vi "Final Project GUI.vi"() -> ()   [LabVIEW 2021]
uses:
  Serial - XON-XOFF Characters.ctl
  Serial - ASCII Characters-1.ctl
  Serial - Settings.ctl
  Lab4/ESP32-PSOC-State Machine.ctl
  <vilib>/Instr/_visa.llb/VISA Flush IO Buffer Mask.ctl
  <vilib>/numeric/Random Number (Range) DBL.vi
  <vilib>/addons/control/pid/pid.llb/PID (DBL).vi
  <vilib>/Instr/_visa.llb/VISA Configure Serial Port (Instr).vi
  <vilib>/picture/picture.llb/Draw True-Color Pixmap.vi
  <vilib>/addons/control/pid/NI_PID_pid.lvlib
  <vilib>/Analysis/NI_AALBase.lvlib
panel:
  out "Actuator Test Chart 4":dbl(graph)
  out "Actuator Test Chart 3":dbl(graph)
  out "Actuator Test Chart 2":dbl(graph)
  in  "Stop 7":bool
  in  "Stop 6":bool
  in  "Stop 5":bool
  out "Actuator Length (inches) 4":string
  out "Actuator Length (inches) 3":string
  out "Actuator Length (inches) 2":string
  out "Actuator Length (inches)":string
  out "Actuator Test Chart":dbl(graph)
  in  "Stop 4":bool
  in  "Termination Character 2":u8=13 format="%.0x"
  in  "End Write on Termination Character? 2":bool=TRUE
  in  "VISA resource name 2":refnum<visa-resource-name>="COM7"
  in  "XON/XOFF Characters 2":T1={"XON"=enum."DC1", "XOFF"=enum."DC3"}
  in  "Serial Settings 2":T3={"baud rate"=115200, "data bits"=8, "parity"=enum."None", "stop bits"=10, "flow control"=0} {"flow control" items=["None"=0, "XON/XOFF"=1, "RTS/CTS"=2, "DTR/DSR"=4]; "stop bits" items=["1.0"=10, "1.5"=15, "2.0"=20]; "data bits" min=5 max=8 step=1; "baud rate" items=["75"=75, "110"=110, "134"=134, "150"=150, "300"=300, "600"=600, "1200"=1200, "1800"=1800, "2400"=2400, "4800"=4800, "7200"=7200, "9600"=9600, "14400"=14400, "19200"=19200, "28800"=28800, "38400"=38400, "56000"=56000, "57600"=57600, "115200"=115200, "128000"=128000, "230400"=230400]}
  in  "End Read on Termination Character? 2":bool=TRUE
  out "Response 3":string
  out "Temperature (deg C)":dbl(graph)
  out "Temperature Histogram":T4(graph)
  in  "Command":string="\n\n"
  in  "Stop 3":bool
  in  "Write":bool
  out "String":string
  out "Response 2":string
  in  "Toggle LED":bool
  in  "Command A":bool
  in  "Command B":bool
  in  "Enum":T5
  out "Connected":bool
  out "error":bool
  out "Read Count":u32=1000
  out "Response":string
  out "Serial Settings:Number of Bytes at Serial Port":u32
  in  "End Read on Termination Character?":bool=TRUE
  in  "Serial Settings":T3={"baud rate"=115200, "data bits"=8, "parity"=enum."None", "stop bits"=10, "flow control"=0} {"flow control" items=["None"=0, "XON/XOFF"=1, "RTS/CTS"=2, "DTR/DSR"=4]; "stop bits" items=["1.0"=10, "1.5"=15, "2.0"=20]; "data bits" min=5 max=8 step=1; "baud rate" items=["75"=75, "110"=110, "134"=134, "150"=150, "300"=300, "600"=600, "1200"=1200, "1800"=1800, "2400"=2400, "4800"=4800, "7200"=7200, "9600"=9600, "14400"=14400, "19200"=19200, "28800"=28800, "38400"=38400, "56000"=56000, "57600"=57600, "115200"=115200, "128000"=128000, "230400"=230400]}
  in  "XON/XOFF Characters":T1={"XON"=enum."DC1", "XOFF"=enum."DC3"}
  in  "VISA resource name":refnum<visa-resource-name>="COM7"
  in  "End Write on Termination Character?":bool=TRUE
  in  "Termination Character":u8=10 format="%.0x"
  in  "Stop 2":bool
  out "Waveform Chart 2":dbl(graph)
  out "Waveform Chart":dbl(graph)
  in  "PID gains":T6={"proportional gain (Kc)"=20.0, "integral time (Ti, min)"=0.008, "derivative time (Td, min)"=0.001} {"derivative time (Td, min)" format="%.3f"; "integral time (Ti, min)" format="%.3f"; "proportional gain (Kc)" format="%.3f"}
  out "2D Picture 2":picture
  out "24-bit pixmap":u32[][](array[numeric]) format="%x"
  out "2D Picture":picture
  in  "Stop":bool
  # "Overview: Demonstrates the use of the VISA functions to write commands to and read responses from a serial instrument continuously in a loop.\nRequirements: NI-VISA Driver\nInstructions:\n1. Using Windows Device Manager take note of the COM port given by Windows to your microcontroller connection\n2. Change the VISA resource name to your COM port from step 1\n3. Run the VI.\n4. Press reset on your microcontroller\n5. Wait for the Ready to accept  Commands message\n6. The sample program response to Command :  T, A, B, I\n7. Specify a Command and click the Write button.\n8 The corresponding response should appear in the Response Window\n9. Click Stop to stop the VI."
  # "CAR"
  # "BONUS ADDITIONS (if time allows)"
types:
  T1 = typedef "Serial - XON-XOFF Characters.ctl" = cluster{"XON":T2, "XOFF":T2}
  T2 = typedef "Serial - ASCII Characters-1.ctl" = enum16{"NUL", "SOH", "STX", "ETX", "EOT", "ENQ", "ACK", "BEL", "BS", "HT", "LF", "VT", "FF", "CR", "SO", "SI", "DLE", "DC1", "DC2", "DC3", "DC4", "NAK", "SYN", "ETB", "CAN", "EM", "SUB", "ESC", "FS", "GS", "RS", "US", "SP", "!", "\"", "#", "$", "%", "&", "'", "(", ")", "*", "+", ",", "- (-)", ".", "/", "0", "1", "2", "3", "4", "5", "6", "7", "8", "9", ":", ";", "<", "=", ">", "?", "@", "A", "B", "C", "D", "E", "F", "G", "H", "I", "J", "K", "L", "M", "N", "O", "P", "Q", "R", "S", "T", "U", "V", "W", "X", "Y", "Z", "[", "\\", "]", "^", "_", "`", "a", "b", "c", "d", "e", "f", "g", "h", "i", "j", "k", "l", "m", "n", "o", "p", "q", "r", "s", "t", "u", "v", "w", "x", "y", "z", "{", "|", "}", "~"}
  T3 = typedef "Serial - Settings.ctl" = cluster{"baud rate":u32, "data bits":u16, "parity":enum16{"None", "Odd", "Even", "Mark", "Space"}, "stop bits":u16, "flow control":u16}
  T4 = cluster{"X Values":dbl[], "Histogram: h(x)":i32[]}
  T5 = typedef "ESP32-PSOC-State Machine.ctl" = enum8{"Init", "Connect", "idle", "send", "wait", "receive", "que", "error", "exit"}
  T6 = cluster{"proportional gain (Kc)":dbl, "integral time (Ti, min)":dbl, "derivative time (Td, min)":dbl}
  T7 = typedef "VISA Flush IO Buffer Mask.ctl" = u16
  T8 = typedef "imagedata.ctl" = cluster{"image type":i32, "image depth":i32, "image":u8[], "mask":u8[], "colors":u32[], "Rectangle":cluster{"left":i16, "top":i16, "right":i16, "bottom":i16}}
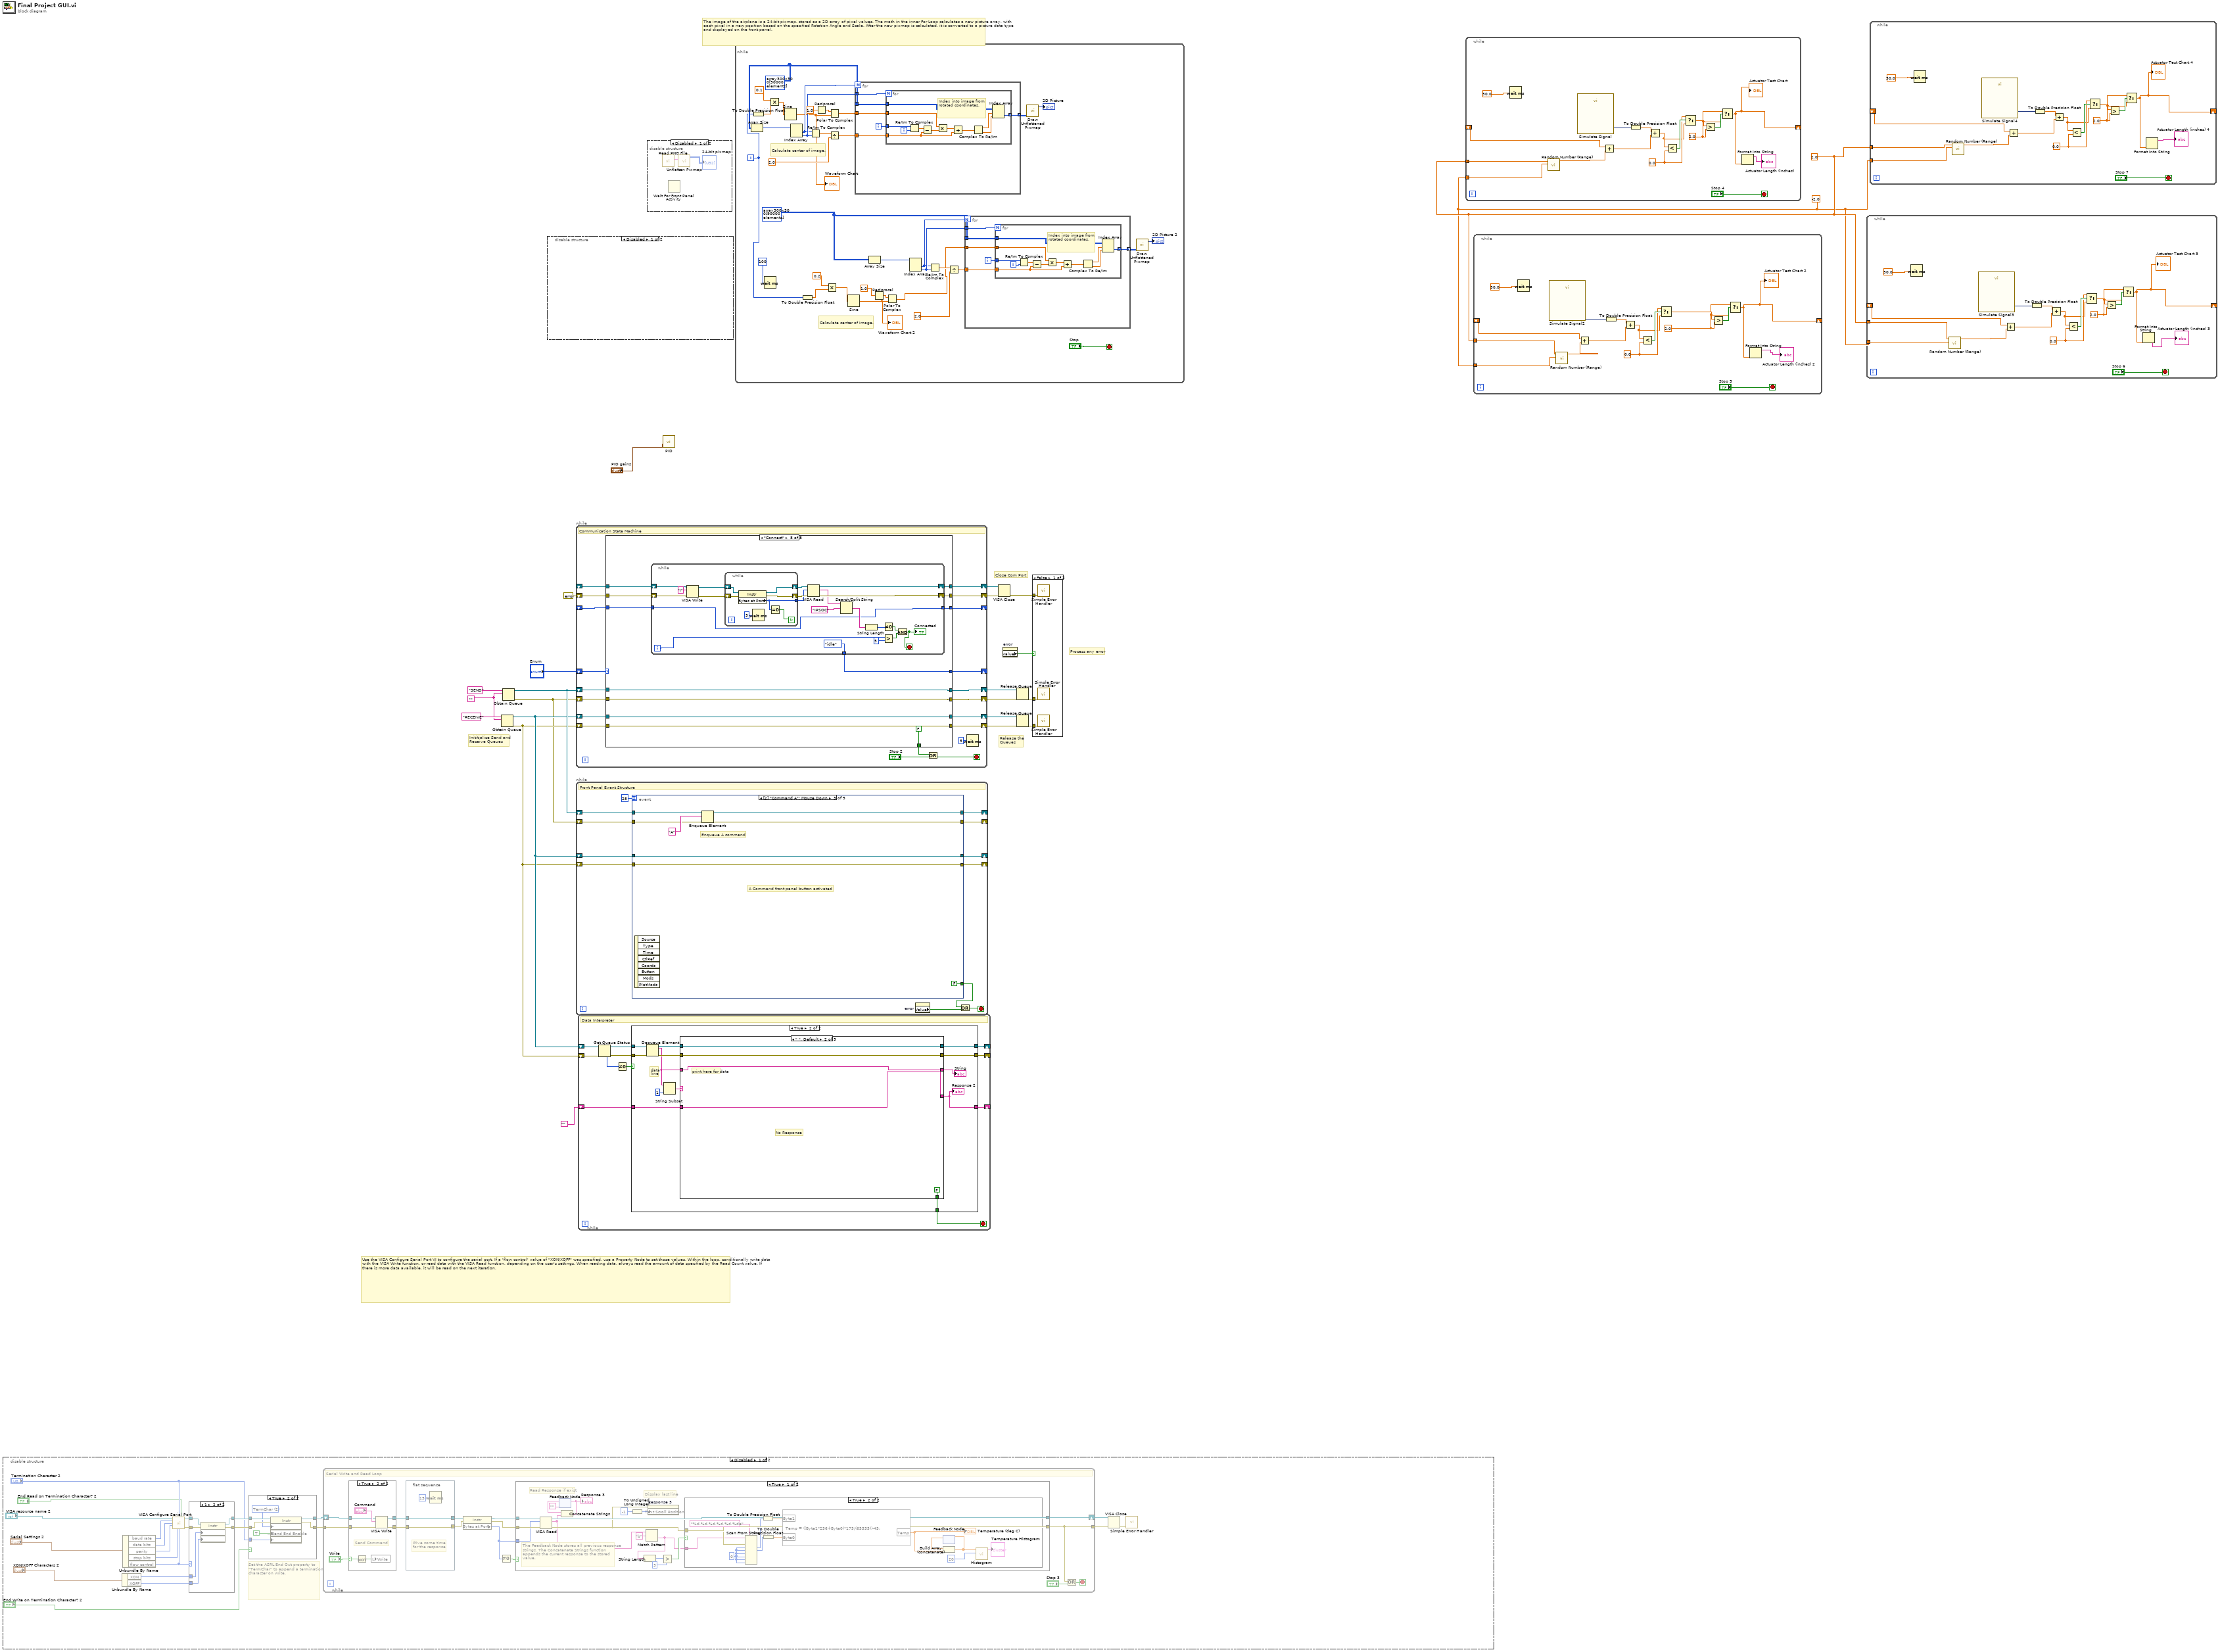
[diagram p0: block diagram]
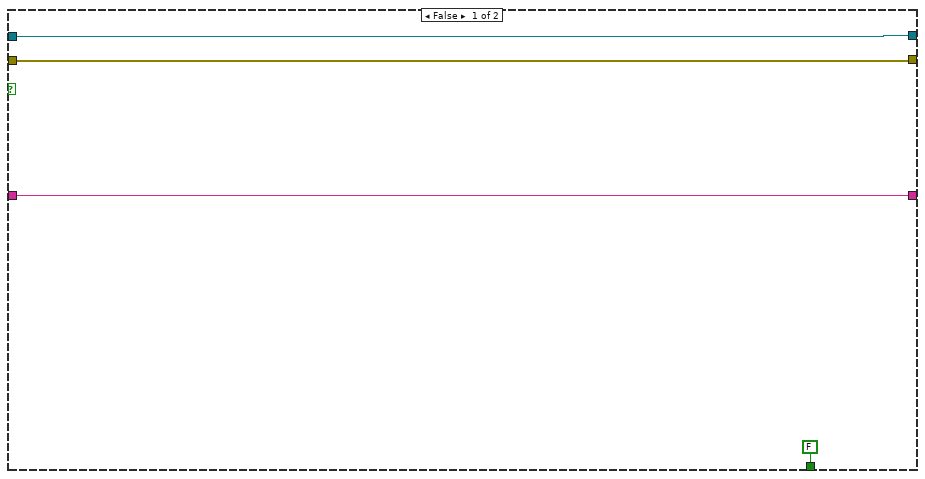
[diagram p9: hidden frame]
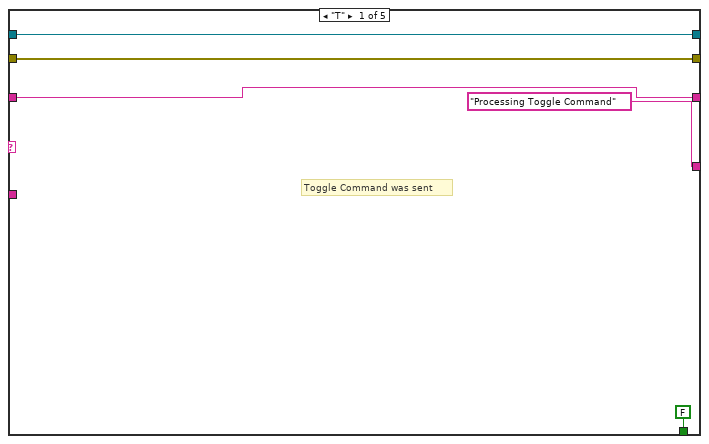
[diagram p10: hidden frame]
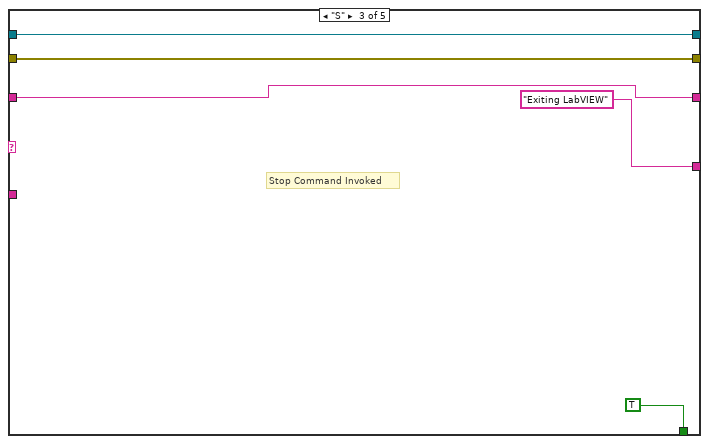
[diagram p11: hidden frame]
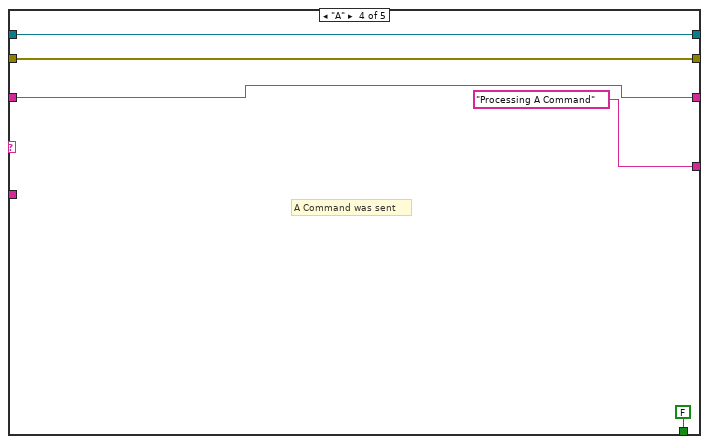
[diagram p12: hidden frame]
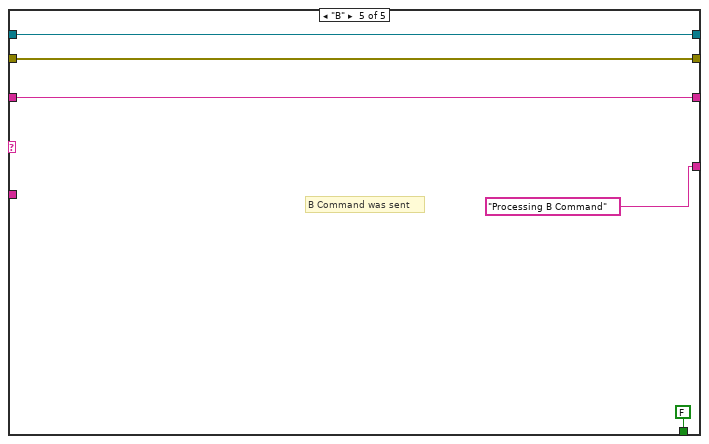
[diagram p13: hidden frame]
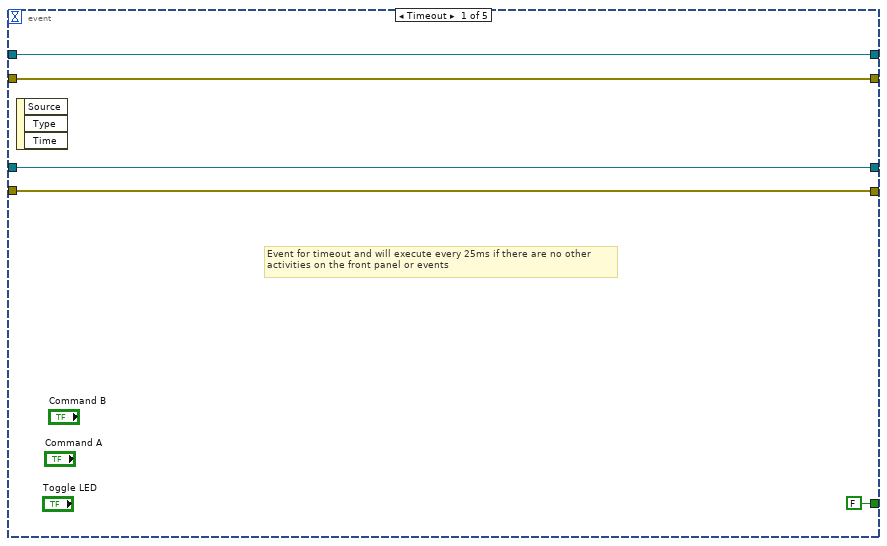
[diagram p14: hidden frame]
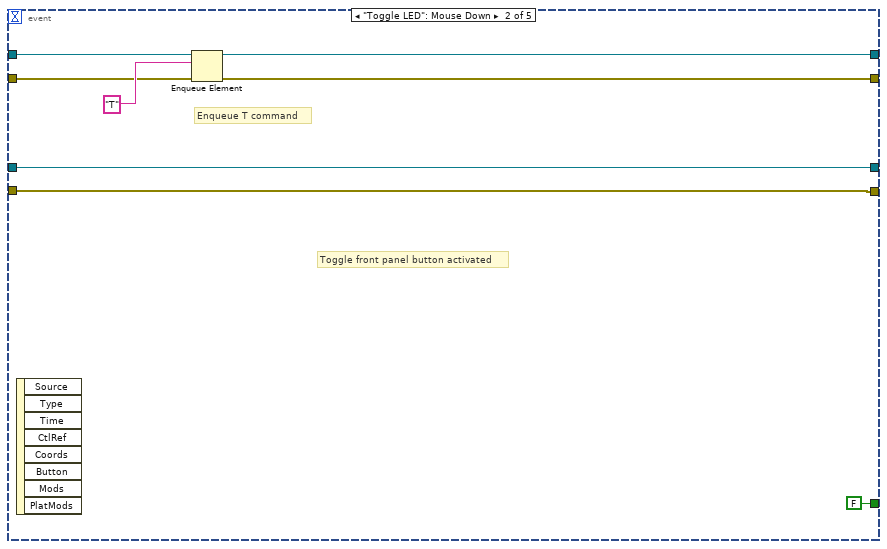
[diagram p15: hidden frame]
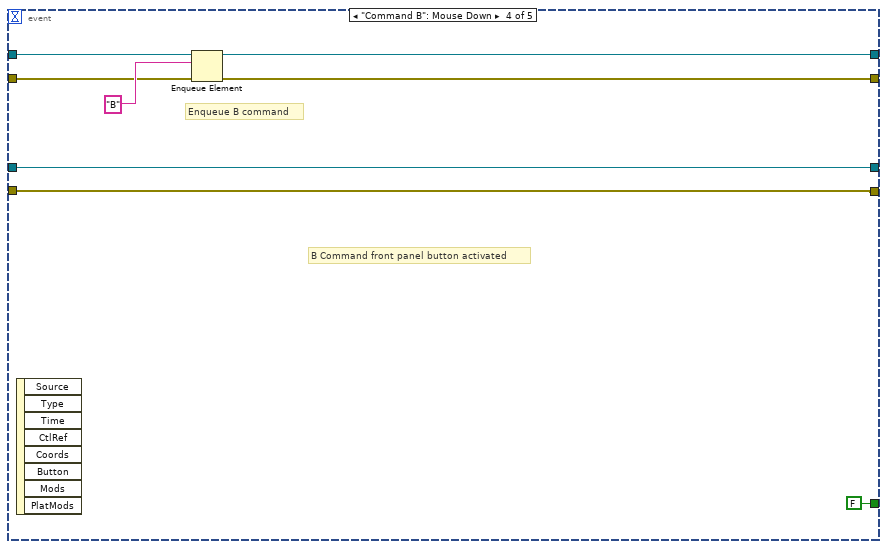
[diagram p16: hidden frame]
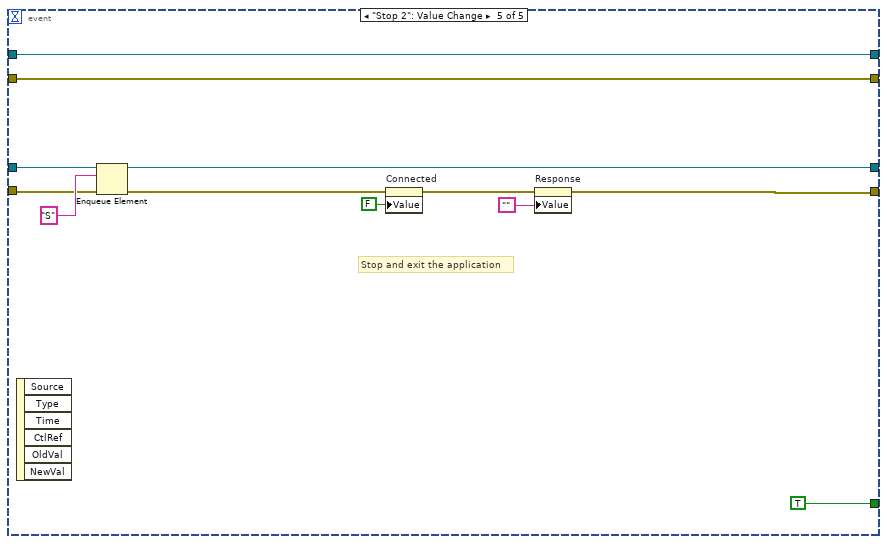
[diagram p17: hidden frame]
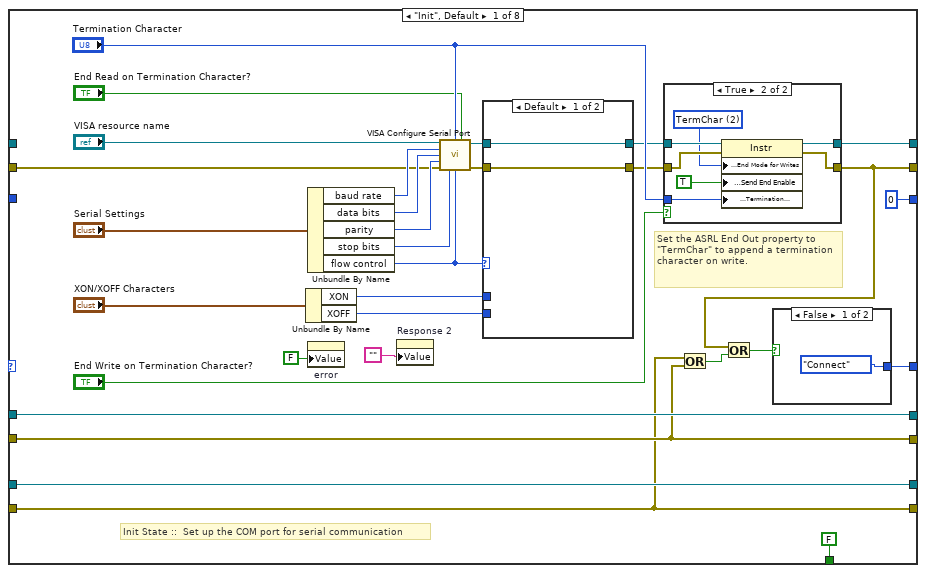
[diagram p18: hidden frame]
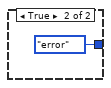
[diagram p19: hidden frame]
diagram:
  w2 = 2.0
  w1 = -2.0
  w12 = ""
  # "Use the VISA Configure Serial Port VI to configure the serial port. If a 'flow control' value of \"XON/XOFF\" was specified, use a Property Node to set those values. Within the loop, conditionally write data with the VISA Write function, or read data with the VISA Read function, depending on the user's settings. When reading data, always read the amount of data specified by the Read Count value. If there is more data available, it will be read on the next iteration."
  # "Process any error"
  # "Release the\nQueues"
  # "Close Com Port"
  # "Inititialize Send and\nReceive Queues"
  # "The image of the airplane is a 24-bit pixmap, stored as a 2D array of pixel values. The math in the inner For Loop calculates a new picture array, with each pixel in a new position based on the specified Rotation Angle and Scale. After the new pixmap is calculated, it is converted to a picture data type and displayed on the front panel."
  n1 = disable-structure shown="Disabled" {
    frame Disabled {
      # "Set the ASRL End Out property to \"TermChar\" to append a termination character on write."
      n2 = Unbundle By Name("XON/XOFF Characters 2") -> ("XON"=w35:T2, "XOFF"=w34:T2)
      n3 = Unbundle By Name("Serial Settings 2") -> ("baud rate"=w40:u32, "data bits"=w41:u16, "parity"=w42:enum16{"None", "Odd", "Even", "Mark", "Space"}, "stop bits"=w43:u16, "flow control"=w36:u16)
      n4 = call-poly "VISA Configure Serial Port"("VISA resource name"="VISA resource name 2", "termination char\n(0xA = '\\n' = LF)"="Termination Character 2", "Enable Termination\nChar (T)"="End Read on Termination Character? 2", "baud rate (9600)"=w40, "data bits (8)"=w41, "parity (0:none)"=w42, "stop bits (10: 1 bit)"=w43, "flow control (0:none)"=w36) -> ("VISA resource name out"=w44:refnum<visa-resource-name>, "error out"=w45:errorcluster)  [unwired: 2 in, 4 out]
      n5 = case shown="1" w36 {
        tunnel: [w55 w62] -> w33
        tunnel: [w56 w61] -> w31
        tunnel: w45 -> [w55 w60]
        tunnel: w44 -> [w56 w59]
        tunnel: w35 -> [_ w58]
        tunnel: w34 -> [_ w57]
        frame Default {
        }
        frame 1 {
          n6 = property class="Instr"(reference=w59, error in=w60, "Serial Settings:Flow Control XON Character"=w58, "Serial Settings:Flow Control XOFF Character"=w57) -> (reference out=w61:refnum<visa-resource-name>, error out=w62:errorcluster)
        }
      }
      n7 = case shown="True" "End Write on Termination Character? 2" {
        tunnel: w31 -> [w46 w54]
        tunnel: w33 -> [w47 w53]
        tunnel: [w46 w52] -> w30
        tunnel: [w47 w51] -> w32
        tunnel: "Termination Character 2" -> [_ w49]
        frame False {
        }
        frame True {
          w50 = u16 2 items=["None", "LastBit", "TermChar", "Break"] ("Serial Settings:Serial End Mode for Writes")
          n8 = property class="Instr"(reference=w54, error in=w53, "Serial Settings:End Mode for Writes"=w50, "Message Based Settings:Send End Enable"=TRUE, "Message Based Settings:Termination Character"=w49) -> (reference out=w52:refnum<visa-resource-name>, error out=w51:errorcluster)
        }
      }
      n9 = while {
        shift-right: [w77] -> w37
        shift-left: w30 -> [w76]
        tunnel: w32 -> [w75]
        tunnel: [w73] -> w38
        stop <- w74 stop-if-true
        # "Serial Write and Read Loop"
        n10 = case shown="True" "Write" {
          selector: "Write" -> [_ w84]
          tunnel: w76 -> [w82 w88]
          tunnel: w75 -> [w81 w87]
          tunnel: [w82 w86] -> w66
          tunnel: [w81 w85] -> w64
          frame False {
          }
          frame True {
            # "Send Command"
            n11 = Not(x=w84) -> (.not. x?=w83:bool)
            n12 = local write "Write"(w83) -> ()
            n13 = VISA Write(VISA resource name=w88, write buffer="Command", error in (no error)=w87) -> (VISA resource name out=w86:refnum<visa-resource-name>, error out=w85:errorcluster)  [unwired: 1 out]
          }
        }
        n14 = flat-sequence {
          tunnel: w66 -> [w80]
          tunnel: [w80] -> w65
          tunnel: w64 -> [w79]
          tunnel: [w79] -> w63
          frame #0 {
            # "Give some time\nfor the response"
            n15 = Wait (ms)(milliseconds to wait=u32 15) -> ()  [unwired: 1 out]
          }
        }
        n16 = property class="Instr"(reference=w65, error in=w63) -> (reference out=w69:refnum<visa-resource-name>, error out=w70:errorcluster, "Bytes at Port"=w67:u32)
        n17 = Not Equal To 0?(x=w67) -> (x != 0?=w68:bool)
        n18 = case shown="True" w68 {
          tunnel: [w99 w120] -> w77
          tunnel: w69 -> [w105 w120]
          tunnel: [w96 w119] -> w73
          tunnel: w70 -> [w104 w119]
          tunnel: w67 -> [w100 _]
          frame True {
            # "Read Response if exist"
            # "Display last line"
            # "The Feedback Node stores all previous response strings. The Concatenate Strings function appends the current response to the stored value."
            n19 = VISA Read(VISA resource name=w105, byte count=w100, error in (no error)=w104) -> (VISA resource name out=w99:refnum<visa-resource-name>, read buffer=w91:string, error out=w96:errorcluster)  [unwired: 1 out]
            n20 = feedback #1("") -> (w103:string)
            n21 = Concatenate Strings(w103, w91) -> (w102:string)
            "Response 3" <- w102
            n22 = feedback-in #1(w102) -> ()
            n23 = To Unsigned Long Integer(number=-1 ("Text.Scroll Position")) -> (unsigned 32bit integer=w97:u32)
            n24 = Match Pattern(string=w91, regular expression="b") -> (after substring=w90:string)  [unwired: 1 in, 3 out]
            n25 = String Length(string=w90) -> (length=w95:i32)
            n26 = property on="Response 3" class="Str"(error in=w96, "Text.Scroll Position"=w97) -> ()  [unwired: 1 in, 2 out]
            n27 = Greater?(x=w95, y=3) -> (0:w93:bool)
            n28 = case shown="True" w93 {
              tunnel: w96 -> [_ w117]
              tunnel: w90 -> [_ w115]
              frame False {
              }
              frame True {
                w118 = u8 0
                n29 = Scan From String(format string="%d,%d,%d,%d,%d,%de", input string=w115, error in=w117, default 1=w118, default 2=w118, default 3=w118, default 4=w118, default 5=w118, default 6=w118) -> (output 1=w114:u8, output 2=w113:u8)  [unwired: 5 in, 3 out]
                n30 = To Double Precision Float(number=w114) -> (double precision float=w112:dbl)
                n31 = To Double Precision Float(number=w113) -> (double precision float=w111:dbl)
                n32 = formula code="Temp = ((Byte1*256+Byte0)*175/(65535))-45;"("Byte1"=w112, "Byte0"=w111) -> ("Temp"=w110:dbl)
                "Temperature (deg C)" <- w110
                n33 = feedback #2() -> (w108:dbl[])  [unwired: 1 in]
                n34 = Build Array (concatenate)(w108, w110) -> (w109:dbl[])
                n35 = feedback-in #2(w109) -> ()
                n36 = call <vilib>:"Histogram.vi"("intervals"=20, "X"=w109) -> ("Histogram Graph"=→"Temperature Histogram":T4)  [unwired: 6 in, 3 out]
              }
            }
          }
          frame False {
          }
        }
        n37 = Or(x=w73, y="Stop 3") -> (x .or. y?=w74:bool)
      }
      n38 = VISA Close(VISA resource name=w37, error in (no error)=w38) -> (error out=w39:errorcluster)
      n39 = call <vilib>:"Simple Error Handler.vi"("error in (no error)"=w39) -> ()  [unwired: 1 in, 8 out]
    }
    frame Enabled {
    }
  }
  n40 = Obtain Queue(name (unnamed)="RECEIVE", element data type=w12) -> (queue out=w11:refnum<queue>, error out=w10:errorcluster)  [unwired: 3 in, 1 out]
  n41 = Obtain Queue(name (unnamed)="SEND", element data type=w12) -> (queue out=w14:refnum<queue>, error out=w4:errorcluster)  [unwired: 3 in, 1 out]
  n42 = disable-structure shown="Disabled" {
    frame Disabled {
    }
    frame Enabled {
    }
  }
  n43 = while {
    shift-right: [w132] -> w22
    shift-left: w14 -> [w140]
    shift-right: [w131] -> w20
    shift-left: w4 -> [w139]
    shift-right: [w130] -> w21
    shift-left: w11 -> [w138]
    shift-right: [w129] -> w17
    shift-left: w10 -> [w137]
    shift-right: [w124] -> _
    shift-left: "Enum" -> [w123]
    shift-right: [w136] -> w16
    shift-left: _ -> [w133]
    shift-right: [w135] -> w15
    shift-left: errorcluster {"status"=FALSE, "code"=0, "source"=""} ("error out") -> [w134]
    shift-right: [w128] -> _
    shift-left: _ -> [w127]
    stop <- w122 stop-if-true
    # "Communication State Machine"
    n44 = case shown="\"Connect\"" w123 {
      selector: w123 -> [_ _ _ _ _ _ w324 _]
      tunnel: [w170 w206 w237 w250 w283 w308 w323 w333] -> w132
      tunnel: [w144 w196 w225 w244 w263 w305 w322 w332] -> w131
      tunnel: [w150 w204 w227 w254 w284 ESP32-PSOC-State_Machine."exit" ("Enum") w324 w329] -> w124
      tunnel: w140 -> [w170 w208 w239 w250 w283 w308 w323 w333]
      tunnel: w139 -> [w144 w207 w238 w244 w263 w305 w322 w332]
      tunnel: w138 -> [w171 w202 w234 w247 w278 w307 w321 w331]
      tunnel: w137 -> [w143 w195 w224 w243 w262 w304 w312 w330]
      tunnel: [w152 w199 w235 w252 w273 w310 w327 w336] -> w136
      tunnel: [w146 w197 w226 w245 w264 w306 w326 w337] -> w135
      tunnel: w134 -> [w148 w198 w230 w251 w266 w306 w326 w338]
      tunnel: w133 -> [_ w200 w232 w253 w281 w310 w327 w339]
      tunnel: [w171 w202 w234 w247 w276 w307 w319 w331] -> w130
      tunnel: [w143 w195 w224 w243 w277 w304 w315 w330] -> w129
      tunnel: [u32 0 ("Bytes at Port") w201 w233 w249 w279 w309 w325 w334] -> w128
      tunnel: w127 -> [_ w201 w233 _ w275 w309 w325 w335]
      tunnel: [FALSE FALSE FALSE FALSE FALSE FALSE TRUE FALSE] -> w121
      frame "Init", Default {
        # "Init State ::  Set up the COM port for serial communication"
        # "Set the ASRL End Out property to \"TermChar\" to append a termination character on write."
        n45 = Unbundle By Name("XON/XOFF Characters") -> ("XON"=w164:T2, "XOFF"=w165:T2)
        n46 = Unbundle By Name("Serial Settings") -> ("baud rate"=w160:u32, "data bits"=w159:u16, "parity"=w158:enum16{"None", "Odd", "Even", "Mark", "Space"}, "stop bits"=w157:u16, "flow control"=w163:u16)
        n47 = property on="error" class="Bool (strict)"("Value"=FALSE ("error")) -> ()  [unwired: 2 in, 2 out]
        n48 = property on="Response 2" class="Str"("Value"="") -> ()  [unwired: 2 in, 2 out]
        n49 = call-poly "VISA Configure Serial Port"("VISA resource name"="VISA resource name", "termination char\n(0xA = '\\n' = LF)"="Termination Character", "Enable Termination\nChar (T)"="End Read on Termination Character?", "baud rate (9600)"=w160, "data bits (8)"=w159, "parity (0:none)"=w158, "error in (no error)"=w148, "stop bits (10: 1 bit)"=w157, "flow control (0:none)"=w163) -> ("VISA resource name out"=w156:refnum<visa-resource-name>, "error out"=w155:errorcluster)  [unwired: 1 in, 4 out]
        n50 = case shown="Default" w163 {
          tunnel: [w183 w192] -> w166
          tunnel: [w184 w191] -> w167
          tunnel: w155 -> [w183 w190]
          tunnel: w156 -> [w184 w189]
          tunnel: w164 -> [_ w188]
          tunnel: w165 -> [_ w187]
          frame Default {
          }
          frame 1 {
            n51 = To Unsigned Byte Integer(number=w187) -> (unsigned 8bit integer=w186:u8)
            n52 = To Unsigned Byte Integer(number=w188) -> (unsigned 8bit integer=w185:u8)
            n53 = property class="Instr"(reference=w189, error in=w190, "Serial Settings:Flow Control XON Character"=w185, "Serial Settings:Flow Control XOFF Character"=w186) -> (reference out=w191:refnum<visa-resource-name>, error out=w192:errorcluster)
          }
        }
        n54 = case shown="True" "End Write on Termination Character?" {
          tunnel: w167 -> [w174 w182]
          tunnel: w166 -> [w175 w181]
          tunnel: [w174 w180] -> w152
          tunnel: [w175 w179] -> w146
          tunnel: "Termination Character" -> [_ w177]
          frame False {
          }
          frame True {
            w178 = u16 2 items=["None", "LastBit", "TermChar", "Break"] ("Serial Settings:Serial End Mode for Writes")
            n55 = property class="Instr"(reference=w182, error in=w181, "Serial Settings:End Mode for Writes"=w178, "Message Based Settings:Send End Enable"=TRUE, "Message Based Settings:Termination Character"=w177) -> (reference out=w180:refnum<visa-resource-name>, error out=w179:errorcluster)
          }
        }
        n56 = Or(x=w143, y=w144) -> (x .or. y?=w145:bool)
        n57 = Or(x=w146, y=w145) -> (x .or. y?=w147:bool)
        n58 = case shown="False" w147 {
          tunnel: [ESP32-PSOC-State_Machine."Connect" ("Enum") ESP32-PSOC-State_Machine."error" ("Enum")] -> w150
          frame False {
          }
          frame True {
          }
        }
      }
      frame "idle" {
        # "Idle State ::  Clear any boot message and wait for command in the queue"
        n59 = Get Queue Status(queue=w208, error in (no error)=w207) -> (queue out=w206:refnum<queue>, error out=w196:errorcluster, # elements in queue=w205:i32)  [unwired: 1 in, 5 out]
        n60 = Not Equal To 0?(x=w205) -> (x != 0?=w203:bool)
        n61 = while {
          tunnel: w200 -> [w221]
          tunnel: [w217] -> w199
          tunnel: w198 -> [w220]
          tunnel: [w215] -> w197
          stop <- w219 continue-if-true
          # "Clearing boot message"
          n62 = property class="Instr"(reference=w221, error in=w220) -> (reference out=w218:refnum<visa-resource-name>, error out=w216:errorcluster, "Serial Settings:Number of Bytes at Serial Port"=w214:u32)
          "Serial Settings:Number of Bytes at Serial Port" <- w214
          n63 = Not Equal To 0?(x=w214) -> (x != 0?=w219:bool)
          n64 = VISA Read(VISA resource name=w218, byte count=w214, error in (no error)=w216) -> (VISA resource name out=w217:refnum<visa-resource-name>, error out=w215:errorcluster)  [unwired: 2 out]
        }
        n65 = Compound Arithmetic op=OR(w197, w196, w195) -> (w194:bool)
        n66 = case shown="False" w194 {
          tunnel: [w210 ESP32-PSOC-State_Machine."error" ("Enum")] -> w204
          tunnel: w203 -> [w209 _]
          frame False {
            n67 = case shown="True" w209 {
              tunnel: [ESP32-PSOC-State_Machine."idle" ("Enum") ESP32-PSOC-State_Machine."send" ("Enum")] -> w210
              frame False {
              }
              frame True {
              }
            }
          }
          frame True {
          }
        }
      }
      frame "send" {
        w228 = T7 64 items=["Flush Receive Buffer"=16, "Write Transmit Buffer to Device"=32, "Flush Receive Buffer (No I/O)"=64, "Flush Transmit Buffer"=128] ("Mask")
        # "Send the command"
        # "Clear the receive buffer for new message"
        n68 = Dequeue Element(queue=w239, error in (no error)=w238) -> (queue out=w237:refnum<queue>, element=w236:string, error out=w225:errorcluster)  [unwired: 1 in, 1 out]
        n69 = VISA Flush I/O Buffer(VISA resource name=w232, mask (16)=w228, error in (no error)=w230) -> (VISA resource name out=w231:refnum<visa-resource-name>, error out=w229:errorcluster)
        n70 = VISA Write(VISA resource name=w231, write buffer=w236, error in (no error)=w229) -> (VISA resource name out=w235:refnum<visa-resource-name>, error out=w226:errorcluster)  [unwired: 1 out]
        n71 = Compound Arithmetic op=OR(w226, w225, w224) -> (w223:bool)
        n72 = case shown="False" w223 {
          tunnel: [ESP32-PSOC-State_Machine."wait" ("Enum") ESP32-PSOC-State_Machine."error" ("Enum")] -> w227
          frame False {
          }
          frame True {
          }
        }
      }
      frame "wait" {
        # "Wait for Response"
        n73 = property class="Instr"(reference=w253, error in=w251) -> (reference out=w252:refnum<visa-resource-name>, error out=w245:errorcluster, "Serial Settings:Number of Bytes at Serial Port"=w249:u32)
        n74 = Not Equal To 0?(x=w249) -> (x != 0?=w248:bool)
        n75 = Compound Arithmetic op=OR(w245, w244, w243) -> (w246:bool)
        n76 = case shown="False" w246 {
          tunnel: [w256 ESP32-PSOC-State_Machine."Connect" ("Enum")] -> w254
          tunnel: w248 -> [w255 _]
          frame False {
            n77 = case shown="False" w255 {
              tunnel: [ESP32-PSOC-State_Machine."receive" ("Enum") ESP32-PSOC-State_Machine."receive" ("Enum")] -> w256
              frame False {
              }
              frame True {
              }
            }
          }
          frame True {
          }
        }
      }
      frame "receive" {
        # "Process Response and Display"
        # "Read Response"
        n78 = VISA Read(VISA resource name=w281, byte count=w275, error in (no error)=w266) -> (VISA resource name out=w274:refnum<visa-resource-name>, read buffer=w269:string, error out=w280:errorcluster)  [unwired: 1 out]
        n79 = String To Byte Array(string=w269) -> (unsigned byte array=w267:u8[])
        n80 = property class="Instr"(reference=w274, error in=w280) -> (reference out=w273:refnum<visa-resource-name>, error out=w265:errorcluster, "Serial Settings:Number of Bytes at Serial Port"=w279:u32)
        n81 = Index Array(array=w267, index=0) -> (element=w271:u8)
        n82 = Not Equal?(x=w271, y=u8 10) -> (x != y?=w268:bool)
        n83 = Not Equal To 0?(x=w279) -> (x != 0?=w282:bool)
        n84 = case shown="True" w268 {
          tunnel: w267 -> [_ w299]
          tunnel: w265 -> [w290 w292]
          tunnel: [w290 w291] -> w264
          frame False {
          }
          frame True {
            n85 = Delete From Array(array=w299, length=1, index=0) -> (array with subset deleted=w296:u8[])  [unwired: 1 out]
            n86 = property on="Response" class="Str"(error in=w292, "Value"="") -> (error out=w294:errorcluster)  [unwired: 1 in, 1 out]
            n87 = Byte Array To String(unsigned byte array=w296) -> (string=w293:string)
            n88 = property on="Response" class="Str"(error in=w294, "Value"=w293) -> (error out=w291:errorcluster)  [unwired: 1 in, 1 out]
          }
        }
        n89 = Compound Arithmetic op=OR(w264, w263, w262) -> (w261:bool)
        n90 = Enqueue Element(queue=w278, element=w269, error in (no error)=w262) -> (queue out=w276:refnum<queue>, error out=w277:errorcluster)  [unwired: 1 in, 1 out]
        n91 = case shown="True" w261 {
          tunnel: [w286 ESP32-PSOC-State_Machine."error" ("Enum")] -> w284
          tunnel: w282 -> [w285 _]
          frame False {
            n92 = case shown="False" w285 {
              tunnel: [ESP32-PSOC-State_Machine."idle" ("Enum") ESP32-PSOC-State_Machine."receive" ("Enum")] -> w286
              frame False {
              }
              frame True {
              }
            }
          }
          frame True {
          }
        }
        "Read Count" <- w275
      }
      frame "error" {
        # "Processing Errors"
        n93 = Build Array(w306, w305, w304) -> (w303:errorcluster[])
        n94 = for {
          tunnel: w303 -> [w311] mode=indexing
          n95 = call <vilib>:"General Error Handler.vi"("error in (no error)"=w311) -> ()  [unwired: 10 in, 5 out]
        }
        "error" <- TRUE ("error")
      }
      frame "exit" {
        # "Stop execution due to error"
        n96 = Enqueue Element(queue=w321, element="S", error in (no error)=w312) -> (queue out=w319:refnum<queue>, error out=w317:errorcluster)  [unwired: 1 in, 1 out]
        n97 = property on="Connected" class="Bool (strict)"(error in=w317, "Value"=FALSE ("Connected")) -> (error out=w316:errorcluster)  [unwired: 1 in, 1 out]
        n98 = property on="Response" class="Str"(error in=w316, "Value"="") -> (error out=w315:errorcluster)  [unwired: 1 in, 1 out]
      }
      frame "Connect" {
        n99 = while {
          shift-right: [w352] -> w337
          shift-left: w338 -> [w359]
          shift-right: [w354] -> w336
          shift-left: w339 -> [w360]
          tunnel: w335 -> [w341]
          tunnel: [w341] -> w334
          tunnel: [ESP32-PSOC-State_Machine."idle" ("Enum")] -> w329
          i -> [w346]
          stop <- w342 stop-if-true
          n100 = VISA Write(VISA resource name=w360, write buffer="I", error in (no error)=w359) -> (VISA resource name out=w356:refnum<visa-resource-name>, error out=w357:errorcluster)  [unwired: 1 out]
          n101 = while {
            shift-right: [w366] -> w353
            shift-left: w357 -> [w367]
            shift-right: [w364] -> w355
            shift-left: w356 -> [w365]
            tunnel: [w361] -> w351
            stop <- w363 continue-if-true
            n102 = property class="Instr"(reference=w365, error in=w367) -> (reference out=w364:refnum<visa-resource-name>, error out=w366:errorcluster, "Bytes at Port"=w361:u32)
            n103 = Wait (ms)(milliseconds to wait=u32 5) -> ()  [unwired: 1 out]
            n104 = Equal To 0?(x=w361) -> (x = 0?=w363:bool)
          }
          n105 = VISA Read(VISA resource name=w355, byte count=w351, error in (no error)=w353) -> (VISA resource name out=w354:refnum<visa-resource-name>, read buffer=w350:string, error out=w352:errorcluster)  [unwired: 1 out]
          n106 = Search/Split String(string=w350, search string/char (-)="IPSOC") -> (match + rest of string=w348:string)  [unwired: 1 in, 2 out]
          n107 = String Length(string=w348) -> (length=w347:i32)
          n108 = Not Equal To 0?(x=w347) -> (x != 0?=w344:bool)
          n109 = Greater?(x=w346, y=5) -> (0:w343:bool)
          n110 = And(x=w344, y=w343) -> (x .and. y?=w342:bool)
          "Connected" <- w342
        }
      }
    }
    n111 = Or(x=w121, y="Stop 2") -> (x .or. y?=w122:bool)
    n112 = Wait (ms)(milliseconds to wait=u32 5) -> ()  [unwired: 1 out]
  }
  n113 = while {
    shift-right: [w376] -> _
    shift-left: w14 -> [w377]
    shift-right: [w375] -> _
    shift-left: w4 -> [w378]
    shift-right: [w371] -> _
    shift-left: w11 -> [w374]
    shift-right: [w372] -> _
    shift-left: w10 -> [w373]
    stop <- w368 stop-if-true
    # "Front Panel Event Structure"
    n114 = event shown="[2] \"Command A\": Mouse Down" {
      selector: _ -> [_ _ _ _ _]
      dyn-events: _ -> [_ _ _ _ _]
      timeout: 25 -> [_ _ _ _ _]
      tunnel: w378 -> [w382 w390 w398 w406 w418]
      tunnel: w377 -> [w383 w392 w400 w408 w419]
      tunnel: [w383 w389 w397 w405 w419] -> w376
      tunnel: [w382 w388 w396 w404 w418] -> w375
      tunnel: [FALSE FALSE FALSE FALSE TRUE] -> w370
      tunnel: w374 -> [w381 w386 w394 w402 w417]
      tunnel: w373 -> [w380 w385 w393 w401 w415]
      tunnel: [w380 w385 w393 w401 w410] -> w372
      tunnel: [w381 w386 w394 w402 w414] -> w371
      event Timeout {
        # "Event for timeout and will execute every 25ms if there are no other\nactivities on the front panel or events"
        n115 = event-data() -> ()  [unwired: 1 in, 3 out]
      }
      event "Toggle LED": Mouse Down {
        # "Enqueue T command"
        # "Toggle front panel button activated"
        n116 = event-data() -> ()  [unwired: 1 in, 8 out]
        n117 = Enqueue Element(queue=w392, element="T", error in (no error)=w390) -> (queue out=w389:refnum<queue>, error out=w388:errorcluster)  [unwired: 1 in, 1 out]
      }
      event "Command A": Mouse Down {
        # "Enqueue A command"
        # "A Command front panel button activated"
        n118 = event-data() -> ()  [unwired: 1 in, 8 out]
        n119 = Enqueue Element(queue=w400, element="A", error in (no error)=w398) -> (queue out=w397:refnum<queue>, error out=w396:errorcluster)  [unwired: 1 in, 1 out]
      }
      event "Command B": Mouse Down {
        # "Enqueue B command"
        # "B Command front panel button activated"
        n120 = event-data() -> ()  [unwired: 1 in, 8 out]
        n121 = Enqueue Element(queue=w408, element="B", error in (no error)=w406) -> (queue out=w405:refnum<queue>, error out=w404:errorcluster)  [unwired: 1 in, 1 out]
      }
      event "Stop 2": Value Change {
        # "Stop and exit the application"
        n122 = event-data() -> ()  [unwired: 1 in, 6 out]
        n123 = Enqueue Element(queue=w417, element="S", error in (no error)=w415) -> (queue out=w414:refnum<queue>, error out=w413:errorcluster)  [unwired: 1 in, 1 out]
        n124 = property on="Connected" class="Bool (strict)"(error in=w413, "Value"=FALSE ("Connected")) -> (error out=w411:errorcluster)  [unwired: 1 in, 1 out]
        n125 = property on="Response" class="Str"(error in=w411, "Value"="") -> (error out=w410:errorcluster)  [unwired: 1 in, 1 out]
      }
    }
    n126 = property on="error" class="Bool (strict)"() -> ("Value"=w369:bool)  [unwired: 2 in, 2 out]
    n127 = Or(x=w370, y=w369) -> (x .or. y?=w368:bool)
  }
  n128 = while {
    shift-right: [w425] -> _
    shift-left: w11 -> [w431]
    shift-right: [w424] -> _
    shift-left: w10 -> [w430]
    shift-right: [w422] -> _
    shift-left: "" -> [w421]
    stop <- w423 stop-if-true
    # "Data Interpreter"
    n129 = Get Queue Status(queue=w431, error in (no error)=w430) -> (queue out=w427:refnum<queue>, error out=w426:errorcluster, # elements in queue=w429:i32)  [unwired: 1 in, 5 out]
    n130 = Not Equal To 0?(x=w429) -> (x != 0?=w428:bool)
    n131 = case shown="True" w428 {
      tunnel: w427 -> [w435 w448]
      tunnel: w426 -> [w434 w447]
      tunnel: [w435 w442] -> w425
      tunnel: [w434 w441] -> w424
      tunnel: [FALSE w440] -> w423
      tunnel: [w432 w438] -> w422
      tunnel: w421 -> [w432 w437]
      frame False {
      }
      frame True {
        # "data\nline"
        n132 = Dequeue Element(queue=w448, error in (no error)=w447) -> (queue out=w446:refnum<queue>, element=w439:string, error out=w445:errorcluster)  [unwired: 1 in, 1 out]
        n133 = String Subset(string=w439, length (rest)=1 ("length (rest)")) -> (substring=w443:string)  [unwired: 1 in]
        n134 = case shown="\" \", Default" w443 {
          tunnel: w446 -> [w453 w458 w463 w468 w473]
          tunnel: w445 -> [w452 w457 w462 w467 w472]
          tunnel: [w453 w458 w463 w468 w473] -> w442
          tunnel: [w452 w457 w462 w467 w472] -> w441
          tunnel: w439 -> [w449 w454 w459 w464 w469]
          tunnel: [FALSE FALSE TRUE FALSE FALSE] -> w440
          tunnel: ["Processing Toggle Command" w455 "Exiting LabVIEW" "Processing A Command" "Processing B Command"] -> w438
          tunnel: w437 -> [_ w455 _ _ _]
          tunnel: [w449 w454 w459 w464 w469] -> w436
          frame "T" {
            # "Toggle Command was sent"
          }
          frame " ", Default {
            # "print here for data"
            # "No Response"
          }
          frame "S" {
            # "Stop Command Invoked"
          }
          frame "A" {
            # "A Command was sent"
          }
          frame "B" {
            # "B Command was sent"
          }
        }
        "Response 2" <- w438
        "String" <- w436
      }
    }
  }
  n135 = disable-structure shown="Disabled" {
    frame Disabled {
      n136 = call <vilib>:"Read PNG File.vi"() -> ("image data"=w475:T8)  [unwired: 9 in, 2 out]
      n137 = Wait For Front Panel Activity() -> ()  [unwired: 3 in, 1 out]
      n138 = call <vilib>:"Unflatten Pixmap.vi"("image data"=w475) -> ("24-bit pixmap"=→"24-bit pixmap":u32[][])  [unwired: 4 in, 6 out]
    }
    frame Enabled {
    }
  }
  n139 = call-poly <vilib>:"PID.vi"("PID gains"="PID gains") -> ()  [unwired: 9 in, 2 out]
  n140 = while {
    i -> [w481]
    stop <- "Stop" stop-if-true
    w483 = u32[][] array300x300[90000 elements] ("24-bit pixmap")
    w489 = u32[][] array300x300[90000 elements] ("24-bit pixmap")
    # "Calculate center of image."
    # "Calculate center of image."
    n141 = Array Size(array=w489) -> (size(s)=w506:i32[])
    n142 = To Double Precision Float(number=w481) -> (double precision float=w499:dbl)
    n143 = Wait (ms)(milliseconds to wait=u32 100) -> ()  [unwired: 1 out]
    n144 = Multiply(x=0.1, y=w499) -> (x*y=w491:dbl)
    n145 = Sine(x=w491) -> (sin(x)=w476:dbl)
    "Waveform Chart" <- w476
    n146 = Index Array(array=w506) -> (element #1=w504:i32, element #2=w505:i32)  [unwired: 2 in]
    n147 = To Double Precision Float(number=w481) -> (double precision float=w482:dbl)
    n148 = Re/Im To Complex(1:w505, 2:w504) -> (0:w507:cdb)
    n149 = Reciprocal(x=1.0) -> (1/x=w508:dbl)
    n150 = Multiply(x=0.2, y=w482) -> (x*y=w485:dbl)
    n151 = Polar To Complex(1:w476, 2:w508) -> (0:w490:cdb)
    n152 = Divide(x=w507, y=2.0) -> (x/y=w503:cdb)
    n153 = Sine(x=w485) -> (sin(x)=w477:dbl)
    "Waveform Chart 2" <- w477
    n154 = for {
      N: w504 -> [_]
      tunnel: w505 -> [w533]
      tunnel: w489 -> [w532]
      tunnel: [w531] -> w510 mode=indexing
      tunnel: w490 -> [w530]
      tunnel: w503 -> [w529]
      i -> [w534]
      n155 = for {
        N: w533 -> [_]
        tunnel: w534 -> [w543]
        tunnel: w532 -> [w546]
        tunnel: [w545] -> w531 mode=indexing
        tunnel: w530 -> [w540]
        tunnel: w529 -> [w535]
        i -> [w544]
        # "Index into image from rotated coordinates."
        n156 = Re/Im To Complex(1:w544, 2:w543) -> (0:w542:cdb)
        n157 = Subtract(x=w542, y=w535) -> (x-y=w541:cdb)
        n158 = Multiply(x=w540, y=w541) -> (x*y=w539:cdb)
        n159 = Add(x=w539, y=w535) -> (x+y=w538:cdb)
        n160 = Complex To Re/Im(x + iy=w538) -> (x=w537:dbl, y=w536:dbl)
        n161 = Index Array(array=w546, index (row)=w537, index (col)=w536) -> (element=w545:u32)
      }
    }
    n162 = Array Size(array=w483) -> (size(s)=w492:i32[])
    n163 = Reciprocal(x=1.0) -> (1/x=w488:dbl)
    n164 = Polar To Complex(1:w477, 2:w488) -> (0:w480:cdb)
    n165 = Index Array(array=w492) -> (element #1=w494:i32, element #2=w495:i32)  [unwired: 2 in]
    n166 = Re/Im To Complex(1:w495, 2:w494) -> (0:w496:cdb)
    n167 = Divide(x=w496, y=2.0) -> (x/y=w493:cdb)
    n168 = for {
      N: w494 -> [_]
      tunnel: w495 -> [w515]
      tunnel: w483 -> [w514]
      tunnel: [w513] -> w498 mode=indexing
      tunnel: w480 -> [w512]
      tunnel: w493 -> [w511]
      i -> [w516]
      n169 = for {
        N: w515 -> [_]
        tunnel: w516 -> [w525]
        tunnel: w514 -> [w528]
        tunnel: [w527] -> w513 mode=indexing
        tunnel: w512 -> [w522]
        tunnel: w511 -> [w517]
        i -> [w526]
        # "Index into image from rotated coordinates."
        n170 = Re/Im To Complex(1:w526, 2:w525) -> (0:w524:cdb)
        n171 = Subtract(x=w524, y=w517) -> (x-y=w523:cdb)
        n172 = Multiply(x=w522, y=w523) -> (x*y=w521:cdb)
        n173 = Add(x=w521, y=w517) -> (x+y=w520:cdb)
        n174 = Complex To Re/Im(x + iy=w520) -> (x=w519:dbl, y=w518:dbl)
        n175 = Index Array(array=w528, index (row)=w519, index (col)=w518) -> (element=w527:u32)
      }
    }
    n176 = call-poly <vilib>:"Draw Unflattened Pixmap.vi"("data (RGB format)"=w510) -> ("new picture"=→"2D Picture":picture)  [unwired: 8 in]
    n177 = call-poly <vilib>:"Draw Unflattened Pixmap.vi"("data (RGB format)"=w498) -> ("new picture"=→"2D Picture 2":picture)  [unwired: 8 in]
  }
  n178 = VISA Close(VISA resource name=w16, error in (no error)=w15) -> (error out=w7:errorcluster)
  n179 = property on="error" class="Bool (strict)"() -> ("Value"=w3:bool)  [unwired: 2 in, 2 out]
  n180 = Release Queue(queue=w22, error in (no error)=w20) -> (error out=w6:errorcluster)  [unwired: 1 in, 2 out]
  n181 = Release Queue(queue=w21, error in (no error)=w17) -> (error out=w5:errorcluster)  [unwired: 1 in, 2 out]
  n182 = case shown="False" w3 {
    tunnel: w7 -> [w549 _]
    tunnel: w6 -> [w548 _]
    tunnel: w5 -> [w547 _]
    frame False {
      n183 = call <vilib>:"Simple Error Handler.vi"("error in (no error)"=w549) -> ()  [unwired: 1 in, 8 out]
      n184 = call <vilib>:"Simple Error Handler.vi"("error in (no error)"=w548) -> ()  [unwired: 1 in, 8 out]
      n185 = call <vilib>:"Simple Error Handler.vi"("error in (no error)"=w547) -> ()  [unwired: 1 in, 8 out]
    }
    frame True {
    }
  }
  n186 = while {
    shift-right: [w553] -> _
    shift-left: _ -> [w556]
    tunnel: w2 -> [w551]
    tunnel: w1 -> [w550]
    stop <- "Stop 4" stop-if-true
    w562 = 0.0
    w558 = 2.0
    n187 = Wait (ms)(milliseconds to wait=50.0) -> ()  [unwired: 1 out]
    n188 = call-poly <vilib>:"Random Number (Range).vi"("lower bound (0)"=w550, "upper bound (100)"=w551) -> ("number"=w554:dbl)  [unwired: 9 in]
    n189 = call "Simulate Signal"() -> ("Square"=w565:dynamicdata)  [unwired: 14 in, 1 out]
    n190 = Add(x=w556, y=w554) -> (x+y=w555:dbl)
    n191 = To Double Precision Float(number=w565) -> (double precision float=w564:dbl)
    n192 = Add(x=w564, y=w555) -> (x+y=w561:dbl)
    n193 = Less?(x=w561, y=w562) -> (x < y?=w563:bool)
    n194 = Select(t=w562, s=w563, f=w561) -> (s? t:f=w559:dbl)
    n195 = Greater?(x=w559, y=w558) -> (0:w560:bool)
    n196 = Select(t=w558, s=w560, f=w559) -> (s? t:f=w553:dbl)
    "Actuator Test Chart" <- w553
    n197 = Format Into String(w553) -> (resulting string=→"Actuator Length (inches)":string)  [unwired: 3 in, 1 out]
  }
  n198 = while {
    shift-right: [w569] -> _
    shift-left: _ -> [w573]
    tunnel: w2 -> [w568]
    tunnel: w1 -> [w567]
    stop <- "Stop 5" stop-if-true
    w579 = 0.0
    w575 = 2.0
    n199 = Wait (ms)(milliseconds to wait=50.0) -> ()  [unwired: 1 out]
    n200 = call "Simulate Signal2"() -> ("Square"=w582:dynamicdata)  [unwired: 14 in, 1 out]
    n201 = call-poly <vilib>:"Random Number (Range).vi"("lower bound (0)"=w567, "upper bound (100)"=w568) -> ("number"=w571:dbl)  [unwired: 9 in]
    n202 = Add(x=w573, y=w571) -> (x+y=w572:dbl)
    n203 = To Double Precision Float(number=w582) -> (double precision float=w581:dbl)
    n204 = Add(x=w581, y=w572) -> (x+y=w578:dbl)
    n205 = Less?(x=w578, y=w579) -> (x < y?=w580:bool)
    n206 = Select(t=w579, s=w580, f=w578) -> (s? t:f=w576:dbl)
    n207 = Greater?(x=w576, y=w575) -> (0:w577:bool)
    n208 = Select(t=w575, s=w577, f=w576) -> (s? t:f=w569:dbl)
    "Actuator Test Chart 2" <- w569
    n209 = Format Into String(w569) -> (resulting string=→"Actuator Length (inches) 2":string)  [unwired: 3 in, 1 out]
  }
  n210 = while {
    shift-right: [w586] -> _
    shift-left: _ -> [w590]
    tunnel: w2 -> [w585]
    tunnel: w1 -> [w584]
    stop <- "Stop 6" stop-if-true
    w596 = 0.0
    w592 = 2.0
    n211 = Wait (ms)(milliseconds to wait=50.0) -> ()  [unwired: 1 out]
    n212 = call-poly <vilib>:"Random Number (Range).vi"("lower bound (0)"=w584, "upper bound (100)"=w585) -> ("number"=w588:dbl)  [unwired: 9 in]
    n213 = call "Simulate Signal3"() -> ("Square"=w599:dynamicdata)  [unwired: 14 in, 1 out]
    n214 = Add(x=w590, y=w588) -> (x+y=w589:dbl)
    n215 = To Double Precision Float(number=w599) -> (double precision float=w598:dbl)
    n216 = Add(x=w598, y=w589) -> (x+y=w595:dbl)
    n217 = Less?(x=w595, y=w596) -> (x < y?=w597:bool)
    n218 = Select(t=w596, s=w597, f=w595) -> (s? t:f=w593:dbl)
    n219 = Greater?(x=w593, y=w592) -> (0:w594:bool)
    n220 = Select(t=w592, s=w594, f=w593) -> (s? t:f=w586:dbl)
    "Actuator Test Chart 3" <- w586
    n221 = Format Into String(w586) -> (resulting string=→"Actuator Length (inches) 3":string)  [unwired: 3 in, 1 out]
  }
  n222 = while {
    shift-right: [w603] -> _
    shift-left: _ -> [w607]
    tunnel: w1 -> [w602]
    tunnel: w2 -> [w601]
    stop <- "Stop 7" stop-if-true
    w613 = 0.0
    w609 = 2.0
    n223 = Wait (ms)(milliseconds to wait=50.0) -> ()  [unwired: 1 out]
    n224 = call-poly <vilib>:"Random Number (Range).vi"("lower bound (0)"=w602, "upper bound (100)"=w601) -> ("number"=w605:dbl)  [unwired: 9 in]
    n225 = call "Simulate Signal4"() -> ("Square"=w616:dynamicdata)  [unwired: 14 in, 1 out]
    n226 = Add(x=w607, y=w605) -> (x+y=w606:dbl)
    n227 = To Double Precision Float(number=w616) -> (double precision float=w615:dbl)
    n228 = Add(x=w615, y=w606) -> (x+y=w612:dbl)
    n229 = Less?(x=w612, y=w613) -> (x < y?=w614:bool)
    n230 = Select(t=w613, s=w614, f=w612) -> (s? t:f=w610:dbl)
    n231 = Greater?(x=w610, y=w609) -> (0:w611:bool)
    n232 = Select(t=w609, s=w611, f=w610) -> (s? t:f=w603:dbl)
    "Actuator Test Chart 4" <- w603
    n233 = Format Into String(w603) -> (resulting string=→"Actuator Length (inches) 4":string)  [unwired: 3 in, 1 out]
  }
